vi "simple.vi"() -> ()   [LabVIEW 2013]
uses:
  lib/libbuddy/bindings/labview/utility_vi/buddy.lvlib
panel:
  out "fw_info out":T1
  out "output cluster":T2
  in  "packet":T2
  out "Count":i32
  in  "timing":cluster{"period":u32, "averaging":u8}={"period"=1000000, "averaging"=0}
  in  "runtime":T3={"dac_power"=1, "dac_ref"=0, "adc_ref"=0, "adc_gain"=0}
  in  "general":T4={"function"=1, "mode"=0, "operation"=1, "queue"=0, "channel_mask"=255, "resolution"=12}
  out "str_serial":string
  out "str_mfr":string
  out "str_product":string
  out "str_index_1":string
  out "handle":u32 format="%x"
  # "CONFIGURATION"
  # "DEVICE INFO"
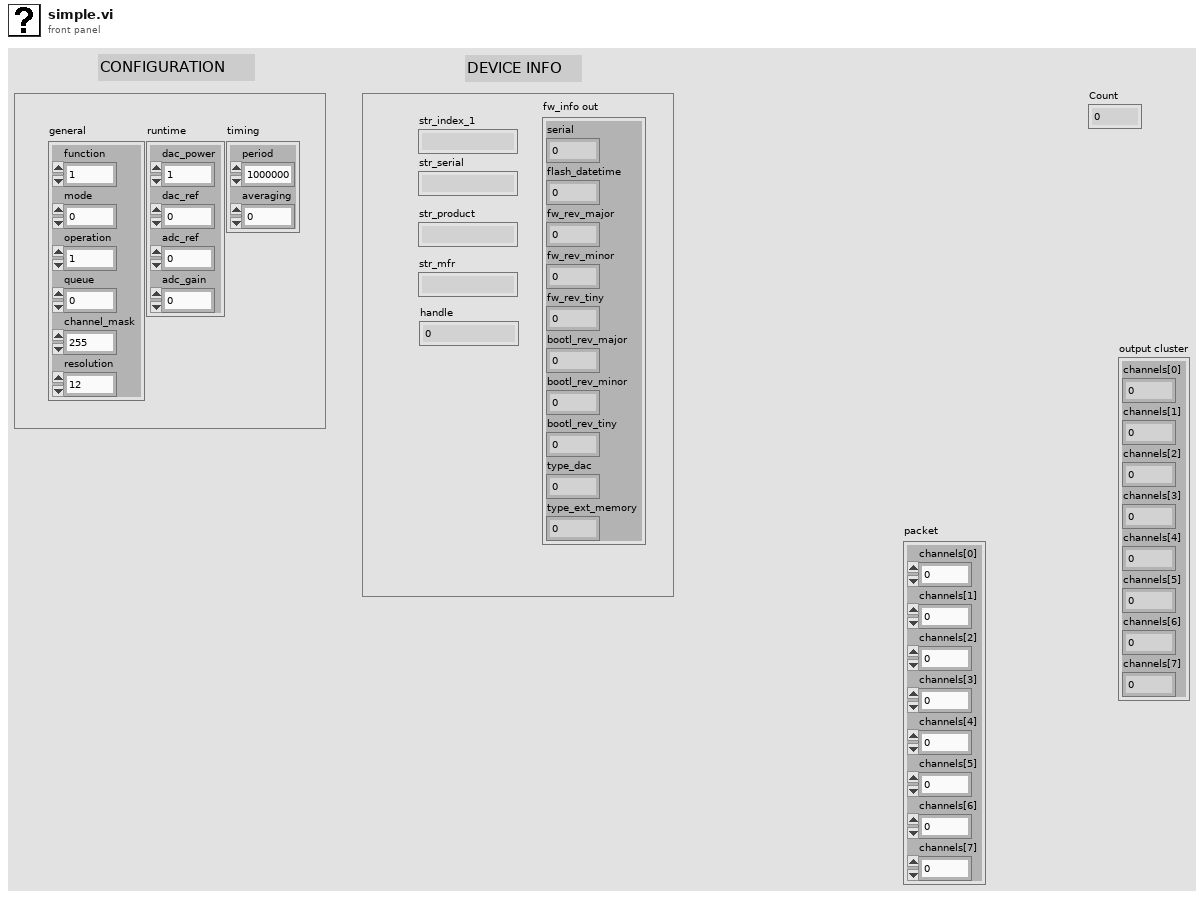
[diagram p1: front panel]
types:
  T1 = cluster{"serial":u32, "flash_datetime":u32, "fw_rev_major":u8, "fw_rev_minor":u8, "fw_rev_tiny":u8, "bootl_rev_major":u8, "bootl_rev_minor":u8, "bootl_rev_tiny":u8, "type_dac":u8, "type_ext_memory":u8}
  T2 = cluster{"channels[0]":u16, "channels[1]":u16, "channels[2]":u16, "channels[3]":u16, "channels[4]":u16, "channels[5]":u16, "channels[6]":u16, "channels[7]":u16}
  T3 = cluster{"dac_power":u8, "dac_ref":u8, "adc_ref":u8, "adc_gain":u8}
  T4 = cluster{"function":u8, "mode":u8, "operation":u8, "queue":u8, "channel_mask":u8, "resolution":u8}
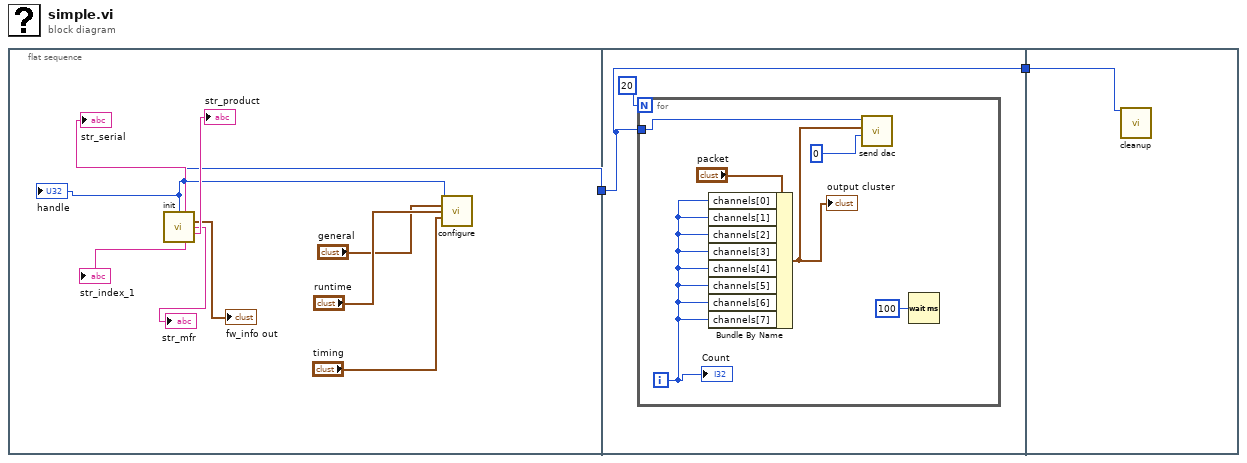
[diagram p0: block diagram]
diagram:
  n1 = flat-sequence {
    tunnel: [w4] -> w2
    tunnel: w2 -> [w12]
    tunnel: [w12] -> w1
    tunnel: w1 -> [w20]
    frame #0 {
      n2 = call "init.vi"() -> ("function return"=w4:u32, "str_serial"=→"str_serial":string, "fw_info out"=→"fw_info out":T1, "str_mfr"=→"str_mfr":string, "str_product"=→"str_product":string, "str_index_1"=→"str_index_1":string)  [unwired: 8 in, 2 out]
      "handle" <- w4
      n3 = call "configure.vi"("handle"=w4, "general"="general", "runtime"="runtime", "timing"="timing") -> ()  [unwired: 6 in, 6 out]
    }
    frame #1 {
      n4 = for {
        N: 20 -> [_]
        tunnel: w12 -> [w17]
        i -> [w15]
        n5 = Bundle By Name(cluster="packet", "channels[0]"=w15, "channels[1]"=w15, "channels[2]"=w15, "channels[3]"=w15, "channels[4]"=w15, "channels[5]"=w15, "channels[6]"=w15, "channels[7]"=w15) -> (w16:T2)
        "output cluster" <- w16
        n6 = call "send dac.vi"("streaming"=0, "packet"=w16, "handle"=w17) -> ()  [unwired: 7 in, 2 out]
        n7 = Wait (ms)(milliseconds to wait=u32 100) -> ()  [unwired: 1 out]
        "Count" <- w15
      }
    }
    frame #2 {
      n8 = call "cleanup.vi"("handle"=w20) -> ()  [unwired: 13 in, 2 out]
    }
  }
